vi "Apply Coefficients SLM.vi"   [LabVIEW 2014]
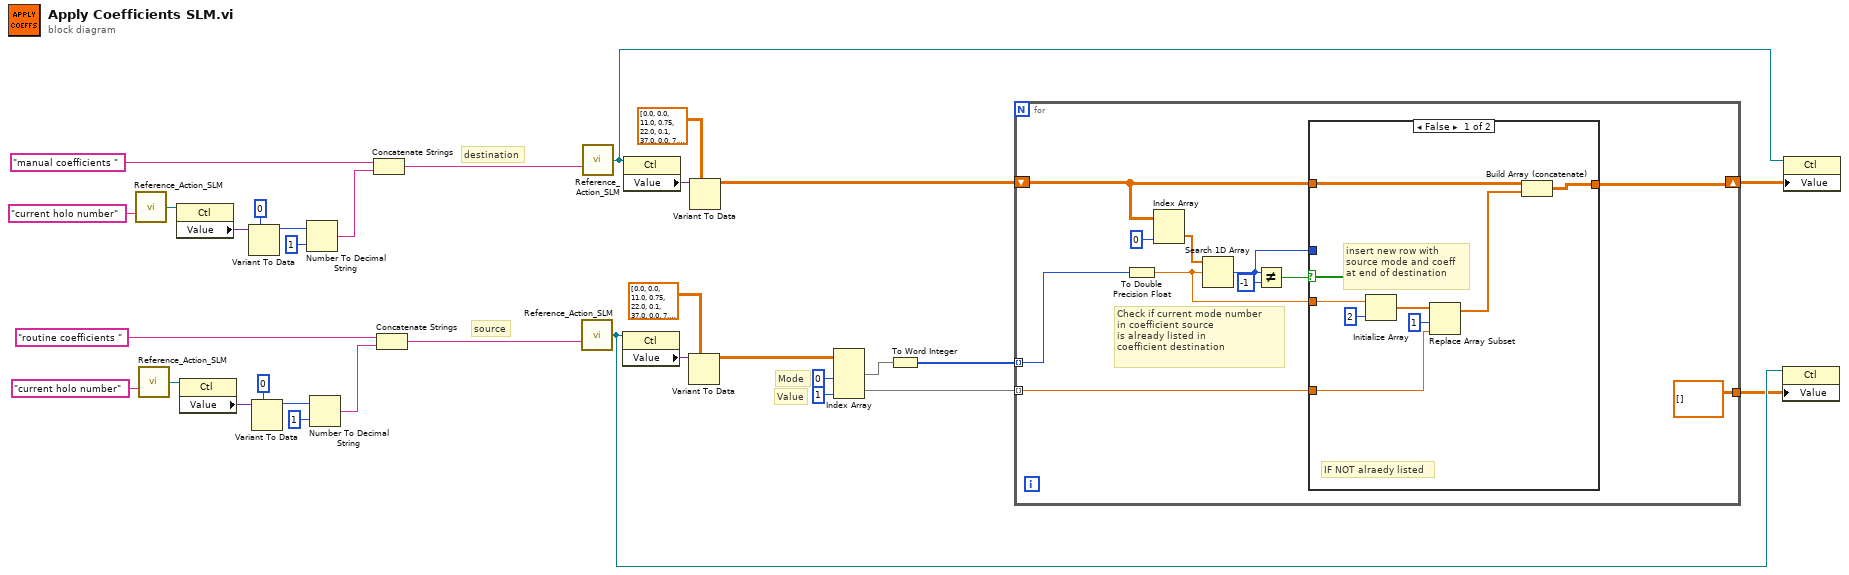
[diagram p0: block diagram]
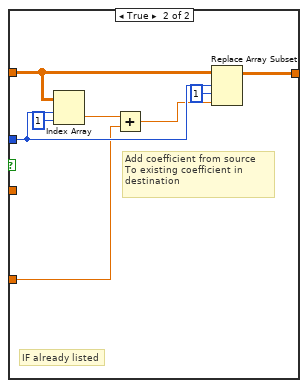
[diagram p2: hidden frame]
diagram:
  # "source"
  # "destination"
  # "Value"
  # "Mode"
  n1 = call "Reference_Action_SLM.vi"("Control Name"="current holo number") -> ("Ref OUT"=w9:refnum<vi>)  [unwired: 12 in, 2 out]
  n2 = call "Reference_Action_SLM.vi"("Control Name"="current holo number") -> ("Ref OUT"=w17:refnum<vi>)  [unwired: 12 in, 2 out]
  n3 = property class="Ctl"(reference=w9) -> ("Value"=w8:variant)  [unwired: 1 in, 2 out]
  n4 = property class="Ctl"(reference=w17) -> ("Value"=w16:variant)  [unwired: 1 in, 2 out]
  n5 = Variant To Data(type=0 ("disabled index (col)"), Variant=w8) -> (data=w6:i32)  [unwired: 1 in, 1 out]
  n6 = Variant To Data(type=0 ("disabled index (col)"), Variant=w16) -> (data=w14:i32)  [unwired: 1 in, 1 out]
  n7 = Number To Decimal String(number=w6, width (-)=i16 1) -> (decimal integer string=w4:string)
  n8 = Number To Decimal String(number=w14, width (-)=i16 1) -> (decimal integer string=w12:string)
  n9 = Concatenate Strings("manual coefficients " ("Control Name"), w4) -> (w1:string)
  n10 = Concatenate Strings("routine coefficients " ("Control Name"), w12) -> (w2:string)
  n11 = call "Reference_Action_SLM.vi"("Control Name"=w2) -> ("Ref OUT"=w20:refnum<vi>)  [unwired: 12 in, 2 out]
  n12 = call "Reference_Action_SLM.vi"("Control Name"=w1) -> ("Ref OUT"=w22:refnum<vi>)  [unwired: 12 in, 2 out]
  n13 = property class="Ctl"(reference=w20) -> ("Value"=w28:variant)  [unwired: 1 in, 2 out]
  n14 = property class="Ctl"(reference=w22) -> ("Value"=w29:variant)  [unwired: 1 in, 2 out]
  n15 = Variant To Data(type=dbl[][] [[0.0, 0.0], [11.0, 0.75], [22.0, 0.1], [37.0, 0.0], [7.0, 0.15], [8.0, 0.1], [5.0, 0.05], [6.0, 0.0], [9.0, 0.0], [10.0, 0.0], [2.0, 0.0], [3.0, -18.3]] ("Mode Coeffs 2"), Variant=w28) -> (data=w26:dbl[][])  [unwired: 1 in, 1 out]
  n16 = Variant To Data(type=dbl[][] [[0.0, 0.0], [11.0, 0.75], [22.0, 0.1], [37.0, 0.0], [7.0, 0.15], [8.0, 0.1], [5.0, 0.05], [6.0, 0.0], [9.0, 0.0], [10.0, 0.0], [2.0, 0.0], [3.0, -18.3]] ("Mode Coeffs 2"), Variant=w29) -> (data=w23:dbl[][])  [unwired: 1 in, 1 out]
  n17 = Index Array(array=w26, index (col) #1=0 ("disabled index (col)"), index (col) #2=1 ("index (col)")) -> (element #1=w31:dbl[], element #2=w30:dbl[])  [unwired: 2 in]
  n18 = To Word Integer(number=w31) -> (16bit integer=w25:i16[])
  n19 = for {
    tunnel: w30 -> [w38] mode=indexing
    tunnel: w25 -> [w36] mode=indexing
    shift-right: [w37] -> w21
    shift-left: w23 -> [w39]
    tunnel: [dbl[][] []] -> w19
    # "Check if current mode number \nin coefficient source\nis already listed in \ncoefficient destination"
    n20 = To Double Precision Float(number=w36) -> (double precision float=w35:dbl)
    n21 = Index Array(array=w39, index (col)=0 ("disabled index (col)")) -> (element=w43:dbl[])  [unwired: 1 in]
    n22 = Search 1D Array(1D array=w43, element=w35) -> (index of element=w40:i32)  [unwired: 1 in]
    n23 = Not Equal?(x=w40, y=-1) -> (x != y?=w41:bool)
    n24 = case shown="False" w41 {
      tunnel: w40 -> [_ w59]
      tunnel: w39 -> [w47 w54]
      tunnel: w38 -> [w48 w56]
      tunnel: [w46 w53] -> w37
      tunnel: w35 -> [w51 _]
      frame False {
        # "insert new row with \nsource mode and coeff\nat end of destination"
        # "IF NOT alraedy listed"
        n25 = Initialize Array(w51, 2 ("dimension size")) -> (w50:dbl[])
        n26 = Replace Array Subset(array=w50, new element=w48, index=1) -> (w45:dbl[])
        n27 = Build Array (concatenate)(w47, w45) -> (w46:dbl[][])
      }
      frame True {
        # "Add coefficient from source\nTo existing coefficient in \ndestination"
        # "IF already listed"
        n28 = Index Array(array=w54, index (row)=w59, index (col)=1 ("disabled index (col)")) -> (element=w57:dbl)
        n29 = Add(x=w57, y=w56) -> (x+y=w55:dbl)
        n30 = Replace Array Subset(array=w54, new element=w55, index (row)=w59, index (col)=1 ("disabled index (col)")) -> (w53:dbl[][])
      }
    }
  }
  n31 = property class="Ctl"(reference=w20, "Value"=w19) -> ()  [unwired: 1 in, 2 out]
  n32 = property class="Ctl"(reference=w22, "Value"=w21) -> ()  [unwired: 1 in, 2 out]
